vi "Handle Last Ack Core.vi"(4 "error in (no error)":errorcluster, 6 "Last Ack":refnum<class "Last Ack.lvclass">, 7 "HIJ Vision Camera App in":refnum<class "HIJ Vision Camera App.lvclass">) -> (0 "error out":errorcluster, 3 "HIJ Vision Camera App out":refnum<class "HIJ Vision Camera App.lvclass">)   [LabVIEW 2014, in "HIJ Vision Camera App.lvlib" / "HIJ Vision Camera App.lvclass"]
doc: "(<B>Filename</B>: Actor Framework.lvlib:Actor.lvclass:Handle Last Ack Core.vi)\n\nDefines how the caller actor responds to the Last Ack message from a nested actor. The Last Ack message is the final message a nested actor sends to its caller before it shuts down. The message contains information about the final state of the nested actor.\n\nBy default, this method does nothing except return any error the nested actor sent. A descendant class may override this method to define behavior."
uses:
  HIJ Vision Camera App.lvclass
  <vilib>/ActorFramework/LastAck/Last Ack.lvclass
  HIJ Vision Camera App Dialog/HIJ Vision Camera App Dialog/HIJ Vision Camera App Dialog.lvclass
  <vilib>/ActorFramework/LastAck/Last Ack.lvclass/Last Ack.ctl
  <vilib>/ActorFramework/Message Enqueuer/Message Enqueuer.lvclass
  HIJ Vision Camera App.lvclass/HIJ Vision Camera App.ctl
  HIJ Vision Application/HIJ Vision Application/HIJ Vision Application.lvclass
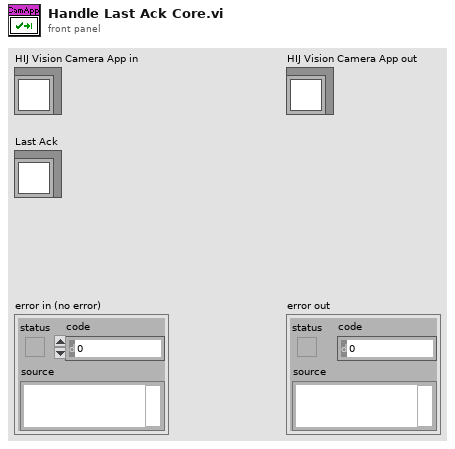
[diagram p1: front panel]
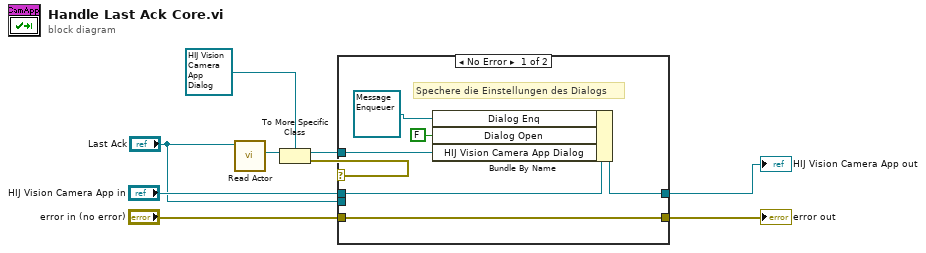
[diagram p0: block diagram]
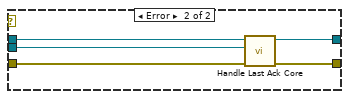
[diagram p2: hidden frame]
diagram:
  n1 = call <vilib>:"Read Actor.vi"("Last Ack"="Last Ack") -> ("Actor"=w3:refnum<class "Actor.lvclass">)  [unwired: 10 in]
  n2 = To More Specific Class(target class=refnum<class "HIJ Vision Camera App Dialog.lvclass"> refnum ("HIJ Vision Camera App Dialog.lvlib:HIJ Vision Camera App Dialog.lvclass"), reference=w3) -> (specific class reference=w2:refnum<class "HIJ Vision Camera App Dialog.lvclass">, error out=w1:errorcluster)  [unwired: 1 in]
  n3 = case shown="No Error" w1 {
    tunnel: [w15 w20] -> w9
    tunnel: [w12 w19] -> w8
    tunnel: "error in (no error)" -> [w15 w18]
    tunnel: "HIJ Vision Camera App in" -> [w14 w17]
    tunnel: "Last Ack" -> [_ w16]
    tunnel: w2 -> [w13 _]
    frame No Error {
      # "Spechere die Einstellungen des Dialogs"
      n4 = Bundle By Name(cluster=w14, "Dialog Enq"=refnum<class "Message Enqueuer.lvclass"> refnum, "Dialog Open"=FALSE, "HIJ Vision Camera App Dialog"=w13) -> (w12:refnum<class "HIJ Vision Camera App.lvclass">)
    }
    frame Error {
      n5 = call-parent "Handle Last Ack Core.vi"("error in (no error)"=w18, "Last Ack"=w16, "Actor in"=w17) -> ("error out"=w20:errorcluster, "Actor out"=w19:refnum<class "HIJ Vision Camera App.lvclass">)  [unwired: 3 in]
    }
  }
  "HIJ Vision Camera App out" <- w8
  "error out" <- w9
